vi "Run.vi"(8 "error in (no error)":errorcluster, 9 "s on last turn":dbl, 10 "Maze (0: Empty, -1: Enemy. >0: Teammate":i32[][](array[numeric]), 11 "Scout In":refnum<class "Coward.lvclass">) -> (0 "error out":errorcluster, 1 "Direction":T1, 2 "Action":T2, 3 "Scout Out":refnum<class "Coward.lvclass">, 4 "Replicated":refnum<class "Square.lvclass">)   [LabVIEW 2015, in "Coward.lvclass"]
uses:
  Coward.lvclass
  Type Defs/Action Enum.ctl
  Type Defs/Direction Enum.ctl
  Square/Square.lvclass
  Formics/Attack Options.ctl
  Coward.lvclass/Coward.ctl
  Common/Common.lvlib
  Formics/Formics.lvclass
  Type Defs/SB Type Defs.lvlib
panel:
  in  "Status":string
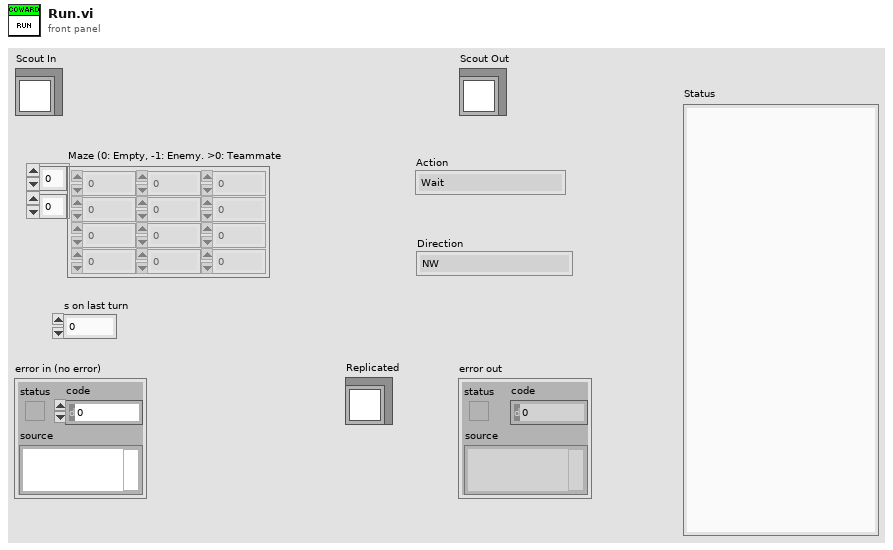
[diagram p1: front panel]
types:
  T1 = typedef "SB Type Defs.lvlib/Direction Enum.ctl" = enum16{"NW", "N", "NE", "E", "SE", "S", "SW", "W"}
  T2 = typedef "SB Type Defs.lvlib/Action Enum.ctl" = enum16{"Wait", "Move", "Attack", "Replicate"}
  T3 = typedef "Formics.lvclass/Attack Options.ctl" = enum16{"Attack", "Run", "Distract"}
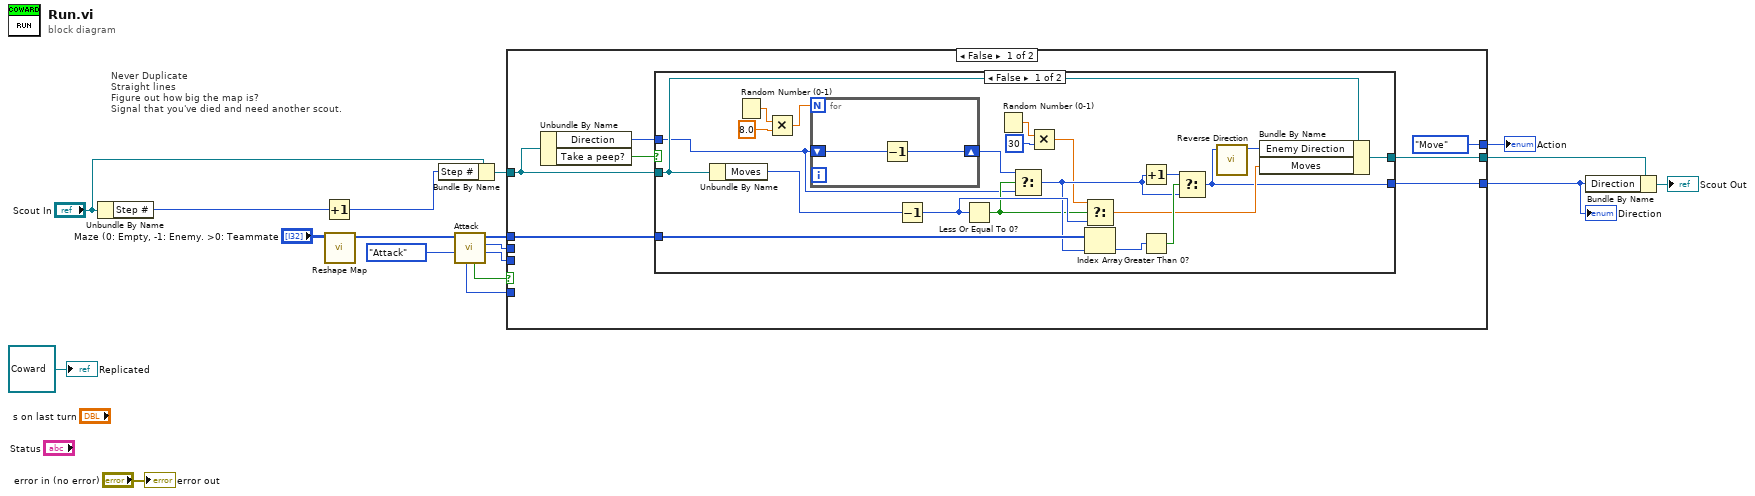
[diagram p0: block diagram]
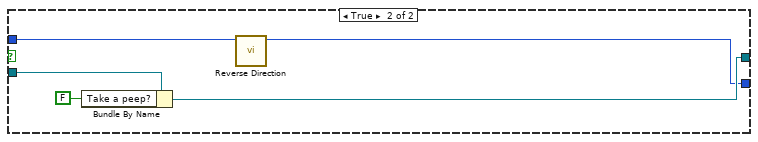
[diagram p2: hidden frame]
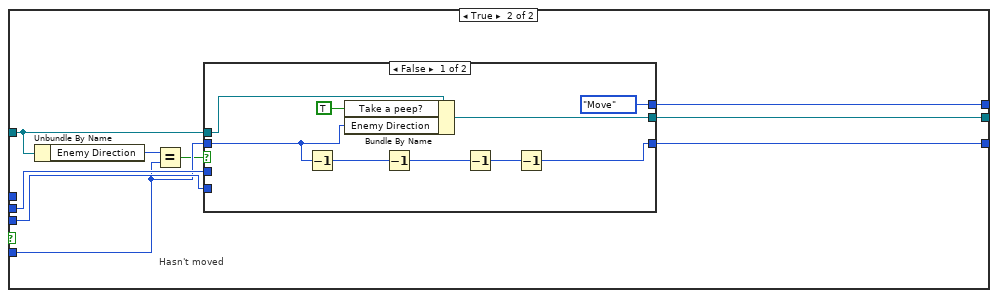
[diagram p3: hidden frame]
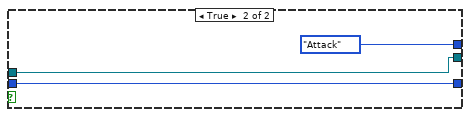
[diagram p4: hidden frame]
diagram:
  # "Never Duplicate\nStraight lines\nFigure out how big the map is?\nSignal that you've died and need another scout."
  n1 = Unbundle By Name("Scout In") -> ("Step #"=w6:i32)
  n2 = Increment(x=w6) -> (x+1=w15:i32)
  n3 = call "Reshape Map.vi"("Maze (0: Empty, -1: Enemy. >0: Teammate"="Maze (0: Empty, -1: Enemy. >0: Teammate") -> ("Map"=w2:i32[])  [unwired: 9 in, 1 out]
  n4 = Bundle By Name(cluster="Scout In", "Step #"=w15) -> (w3:refnum<class "Coward.lvclass">)
  n5 = call "Attack.vi"("Attack?"=Attack_Options."Attack", "Maze (0: Empty, -1: Enemy. >0: Teammate"=w2) -> ("Direction"=w8:i32, "Action"=w10:T2, "Maze (0: Empty, -1: Enemy. >0: Teammate 2"=w1:i32[], "Enemy Found?"=w11:bool, "Enemy Direction"=w4:i32)  [unwired: 4 in, 1 out]
  n6 = case shown="False" w11 {
    tunnel: w10 -> [_ w59]
    tunnel: [Action_Enum."Move" ("Action") w58] -> w9
    tunnel: w8 -> [_ w60]
    tunnel: [w24 w57] -> w7
    tunnel: w1 -> [w23 _]
    tunnel: w3 -> [w20 w61]
    tunnel: [w19 w62] -> w5
    tunnel: w4 -> [_ w55]
    frame False {
      n7 = Unbundle By Name(w20) -> ("Direction"=w22:T1, "Take a peep?"=w21:bool)
      n8 = case shown="False" w21 {
        tunnel: [w26 w49] -> w24
        tunnel: w23 -> [w46 _]
        tunnel: w22 -> [w32 w50]
        tunnel: w20 -> [w41 w53]
        tunnel: [w42 w52] -> w19
        frame False {
          n9 = Unbundle By Name(w41) -> ("Moves"=w40:i32)
          n10 = Random Number (0-1)() -> (number: 0 to 1=w37:dbl)
          n11 = Multiply(x=w37, y=8.0) -> (x*y=w33:dbl)
          n12 = for {
            N: w33 -> [_]
            shift-right: [w47] -> w31
            shift-left: w32 -> [w48]
            n13 = Decrement(x=w48) -> (x-1=w47:T1)
          }
          n14 = Decrement(x=w40) -> (x-1=w38:i32)
          n15 = Less Or Equal To 0?(x=w38) -> (x <= 0?=w34:bool)
          n16 = Random Number (0-1)() -> (number: 0 to 1=w30:dbl)
          n17 = Select(t=w31, s=w34, f=w32) -> (s? t:f=w35:T1)
          n18 = Multiply(x=w30, y=30 ("t")) -> (x*y=w28:dbl)
          n19 = Select(t=w28, s=w34, f=w38) -> (s? t:f=w39:dbl)
          n20 = Index Array(array=w46, index=w35) -> (element=w45:i32)
          n21 = Increment(x=w35) -> (x+1=w43:T1)
          n22 = Greater Than 0?(x=w45) -> (x > 0?=w44:bool)
          n23 = Select(t=w43, s=w44, f=w35) -> (s? t:f=w26:T1)
          n24 = call "Reverse Direction.vi"("Direction"=w26) -> ("Numeric"=w27:i32)  [unwired: 10 in]
          n25 = Bundle By Name(cluster=w41, "Enemy Direction"=w27, "Moves"=w39) -> (w42:refnum<class "Coward.lvclass">)
        }
        frame True {
          n26 = Bundle By Name(cluster=w53, "Take a peep?"=FALSE) -> (w52:refnum<class "Coward.lvclass">)
          n27 = call "Reverse Direction.vi"("Direction"=w50) -> ("Numeric"=w49:i32)  [unwired: 10 in]
        }
      }
    }
    frame True {
      # "Hasn't moved"
      n28 = Unbundle By Name(w61) -> ("Enemy Direction"=w56:T1)
      n29 = Equal?(x=w56, y=w55) -> (x = y?=w54:bool)
      n30 = case shown="False" w54 {
        tunnel: [w71 w74] -> w62
        tunnel: w61 -> [w69 w74]
        tunnel: w60 -> [_ _]
        tunnel: w59 -> [_ _]
        tunnel: [Action_Enum."Move" ("Action") Action_Enum."Attack" ("Action")] -> w58
        tunnel: [w64 w72] -> w57
        tunnel: w55 -> [w65 w72]
        frame False {
          n31 = Decrement(x=w65) -> (x-1=w68:i32)
          n32 = Bundle By Name(cluster=w69, "Take a peep?"=TRUE, "Enemy Direction"=w65) -> (w71:refnum<class "Coward.lvclass">)
          n33 = Decrement(x=w68) -> (x-1=w66:i32)
          n34 = Decrement(x=w66) -> (x-1=w67:i32)
          n35 = Decrement(x=w67) -> (x-1=w64:i32)
        }
        frame True {
        }
      }
    }
  }
  "Action" <- w9
  "Direction" <- w7
  n36 = Bundle By Name(cluster=w5, "Direction"=w7) -> (→"Scout Out":refnum<class "Coward.lvclass">)
  "error out" <- "error in (no error)"
  "Replicated" <- refnum<class "Coward.lvclass"> refnum ("Replicated")
